vi "write to event log.vi"(1 "log file ref":refnum<file>, 2 "time":dbl, 3 "input string":string) -> ()   [LabVIEW 2014]
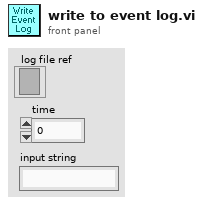
[diagram p1: front panel]
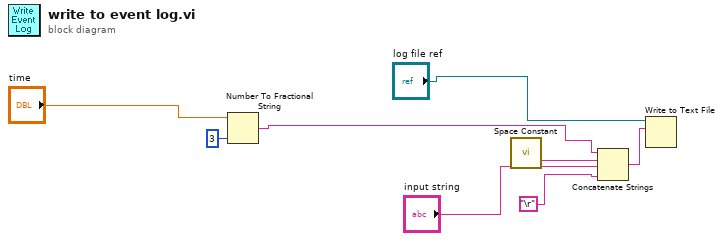
[diagram p0: block diagram]
diagram:
  n1 = Number To Fractional String(number="time", precision (6)=i16 3) -> (F-format string=w2:string)  [unwired: 2 in]
  n2 = call <vilib>:"Space Constant.vi"() -> ("String"=w4:string)
  n3 = Concatenate Strings(w2, w4, "input string", "\r") -> (w5:string)
  n4 = Write to Text File(file (use dialog)="log file ref", text=w5) -> ()  [unwired: 2 in, 3 out]
